vi "Add Context.vi"(7 "Context":string, 9 "MultiErrors in":refnum<class "MultiErrors.lvclass">) -> (1 "Original Context":refnum<class "MultiErrors.lvclass">, 3 "Added Context":refnum<class "MultiErrors.lvclass">)   [LabVIEW 2020, in "VolatusErrorUtilities.lvlib" / "MultiErrors.lvclass"]
uses:
  MultiErrors.lvclass
  MultiErrors.lvclass/MultiErrors.ctl
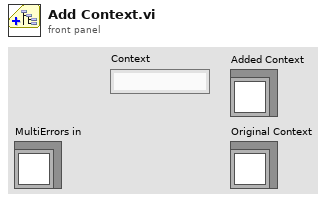
[diagram p1: front panel]
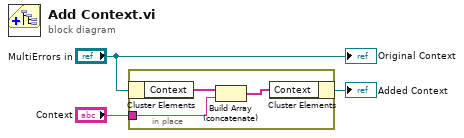
[diagram p0: block diagram]
diagram:
  n1 = in-place {
    in-place-border: "Context" -> [w5]
    n2 = in-place-cluster #1("MultiErrors in") -> ("Context"=w6:string[])
    n3 = Build Array (concatenate)(w6, w5) -> (w4:string[])
    n4 = in-place-cluster #1("Context"=w4) -> (→"Added Context":refnum<class "MultiErrors.lvclass">)
  }
  "Original Context" <- "MultiErrors in"
